vi "Drive_Execute.vi"() -> ()   [LabVIEW 2020]
uses:
  Drive_Control_States.ctl
  Drive_Cluster.ctl
  Drive_Orientation_States.ctl
  Globals/Drive_Globals.vi
  Globals/Sensor_Values.vi
  Globals/Calibration_And_Constant_Globals.vi
panel:
  in  "Back_Right_PID":T1(array[cluster])=[{"Kp"=0.0028, "Ki"=0.0, "Kd"=0.0, "N-Diff"=10, "N-Int"=10, "Int Error Window"=20.0, "Max Ouput"=0.5, "Min Output"=-0.5}, {"Kp"=0.0028, "Ki"=0.0, "Kd"=0.0, "N-Diff"=10, "N-Int"=10, "Int Error Window"=20.0, "Max Ouput"=0.5, "Min Output"=-0.5}]
  in  "Back_Left_PID":T1(array[cluster])=[{"Kp"=0.0028, "Ki"=0.0, "Kd"=0.0, "N-Diff"=10, "N-Int"=10, "Int Error Window"=20.0, "Max Ouput"=0.5, "Min Output"=-0.5}, {"Kp"=0.0028, "Ki"=0.0, "Kd"=0.0, "N-Diff"=10, "N-Int"=10, "Int Error Window"=20.0, "Max Ouput"=0.5, "Min Output"=-0.5}]
  in  "Front_Left_PID":T1(array[cluster])=[{"Kp"=0.0028, "Ki"=0.0, "Kd"=0.0, "N-Diff"=10, "N-Int"=10, "Int Error Window"=20.0, "Max Ouput"=0.5, "Min Output"=-0.5}, {"Kp"=0.0028, "Ki"=0.0, "Kd"=0.0, "N-Diff"=10, "N-Int"=10, "Int Error Window"=20.0, "Max Ouput"=0.5, "Min Output"=-0.5}]
  in  "Front_Right_PID":T1(array[cluster])=[{"Kp"=0.0028, "Ki"=0.0, "Kd"=0.0, "N-Diff"=10, "N-Int"=10, "Int Error Window"=20.0, "Max Ouput"=0.5, "Min Output"=-0.5}, {"Kp"=0.0028, "Ki"=0.0, "Kd"=0.0, "N-Diff"=10, "N-Int"=10, "Int Error Window"=20.0, "Max Ouput"=0.5, "Min Output"=-0.5}]
  out "angles":T2(graph)={"Front_Right"=176.5765625, "Front_ Left"=-4.482062499999984, "Back_Left"=-3.867593749999969, "Back_Right"=175.781515625}
  out "Front_Right":T3(graph)={"Command"=0.010270312500000017, "Proportional"=0.010270312500000017, "Integral"=0.0, "Derivative"=0.0, "Goal"=3.4234375000000057}
  out "Back_Right":T3(graph)={"Command"=0.01265545312500001, "Proportional"=0.01265545312500001, "Integral"=0.0, "Derivative"=0.0, "Goal"=4.218484375000003}
  out "Back_Left":T3(graph)={"Command"=0.011602781249999907, "Proportional"=0.011602781249999907, "Integral"=0.0, "Derivative"=0.0, "Goal"=3.867593749999969}
  out "Front_Left":T3(graph)={"Command"=0.013446187499999951, "Proportional"=0.013446187499999951, "Integral"=0.0, "Derivative"=0.0, "Goal"=4.482062499999984}
  in  "Manual_Target_Angle (deg)":dbl
  in  "Front_Panel_Control":bool
  in  "Hysteresis (deg)":dbl=10.0 format="%#_13g"
  # "0th index alpha,\n1st index beta"
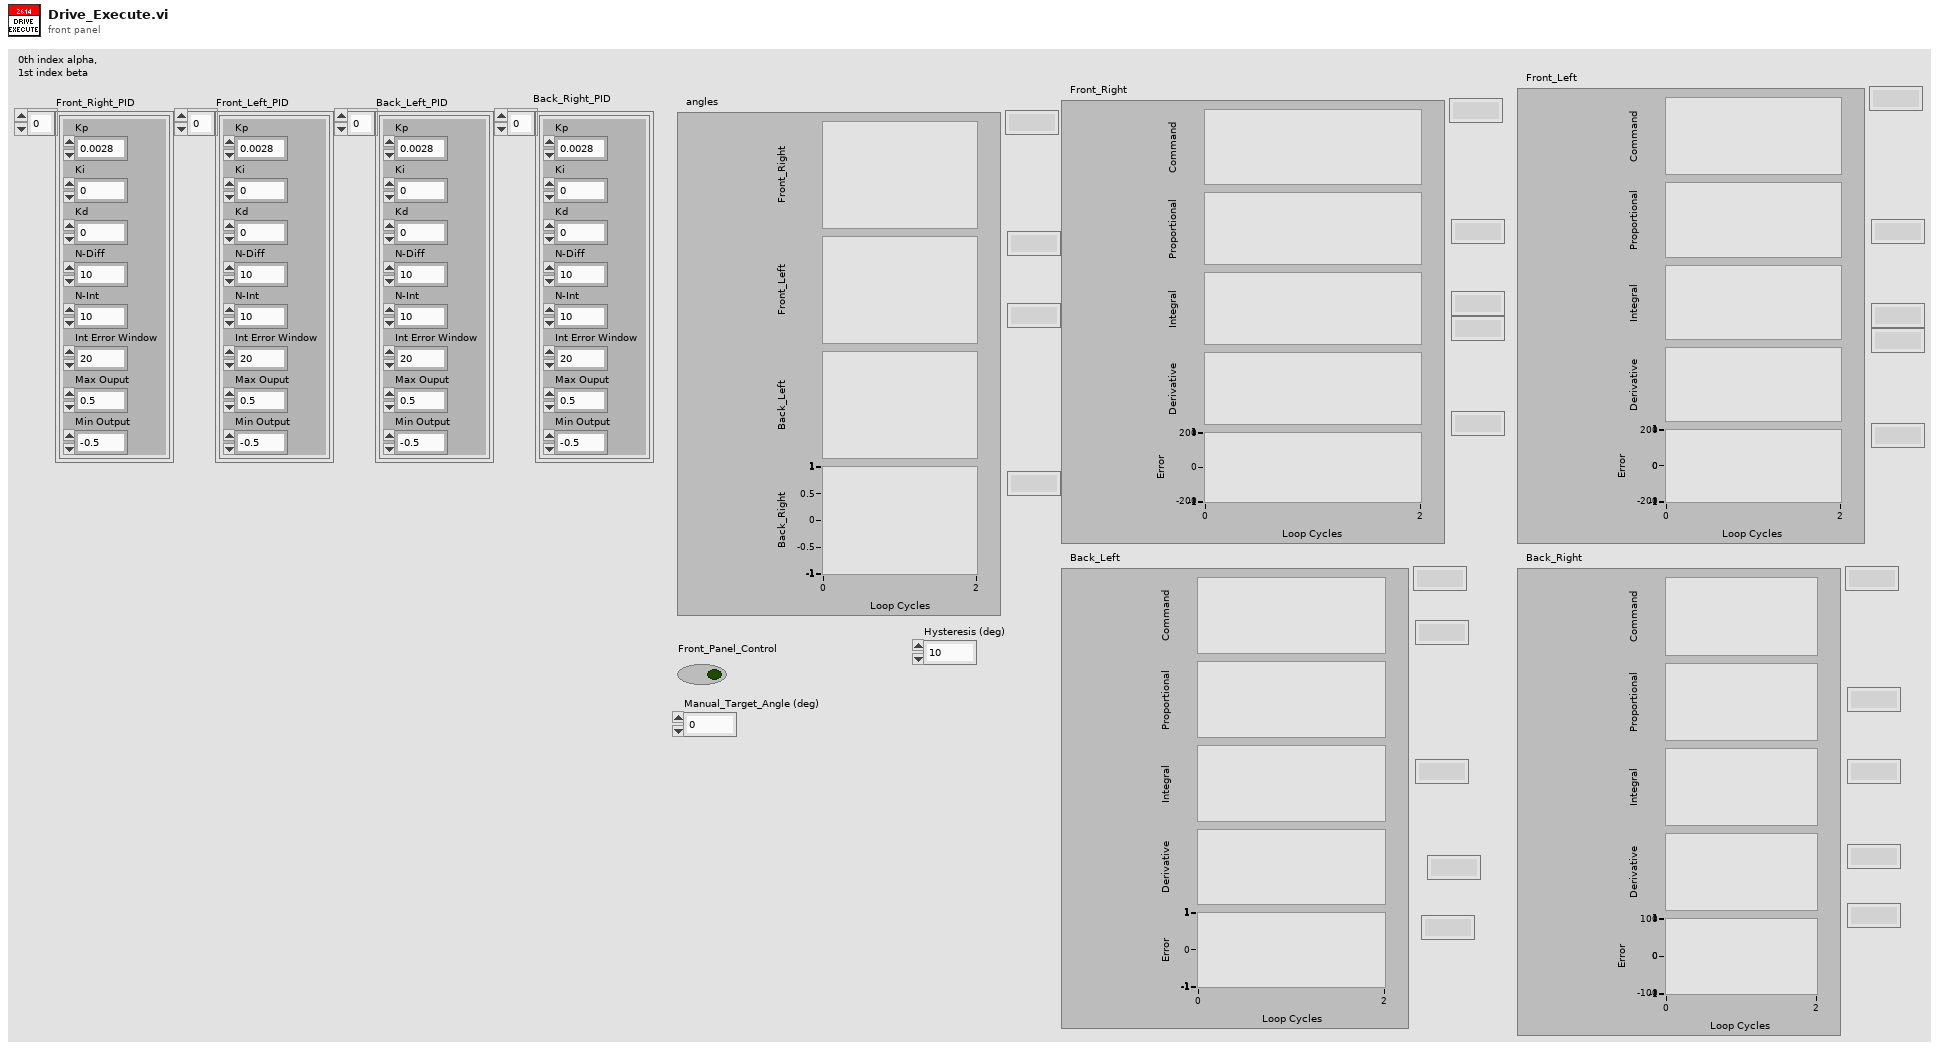
[diagram p1: front panel]
types:
  T1 = cluster{"Kp":dbl, "Ki":dbl, "Kd":dbl, "N-Diff":i32, "N-Int":i32, "Int Error Window":dbl, "Max Ouput":dbl, "Min Output":dbl}[]
  T2 = cluster{"Front_Right":dbl, "Front_ Left":dbl, "Back_Left":dbl, "Back_Right":dbl}
  T3 = cluster{"Command":dbl, "Proportional":dbl, "Integral":dbl, "Derivative":dbl, "Goal":dbl}
  T4 = typedef "Drive_Control_States.ctl" = enum16{"No-Op", "Manual_Control", "Command_DriveDistanceAtAngle", "Command_DrivePath", "Command_SetRobotPose", "Command_Rotate", "Go_To_X"}
  T5 = typedef "Drive_Cluster.ctl" = cluster{"Control_State":T4, "Vertical_Throttle":dbl, "Lateral_Throttle":dbl, "Rotational_Throttle":dbl, "Strafe_In_Deadband":bool, "Rotation_In_Deadband":bool, "Orientation_State":T6, "Parameters":dbl[], "Step":i32, "Auto_Notifier":refnum<notifier>, "PathName":string}
  T6 = typedef "Drive_Orientation_States.ctl" = enum16{"Robot-Oriented", "Field-Oriented"}
  T7 = cluster{"Kp":dbl, "Ki":dbl, "Kd":dbl, "N-Diff":i32, "N-Int":i32, "Int Error Window":dbl, "Max Ouput":dbl, "Min Output":dbl}
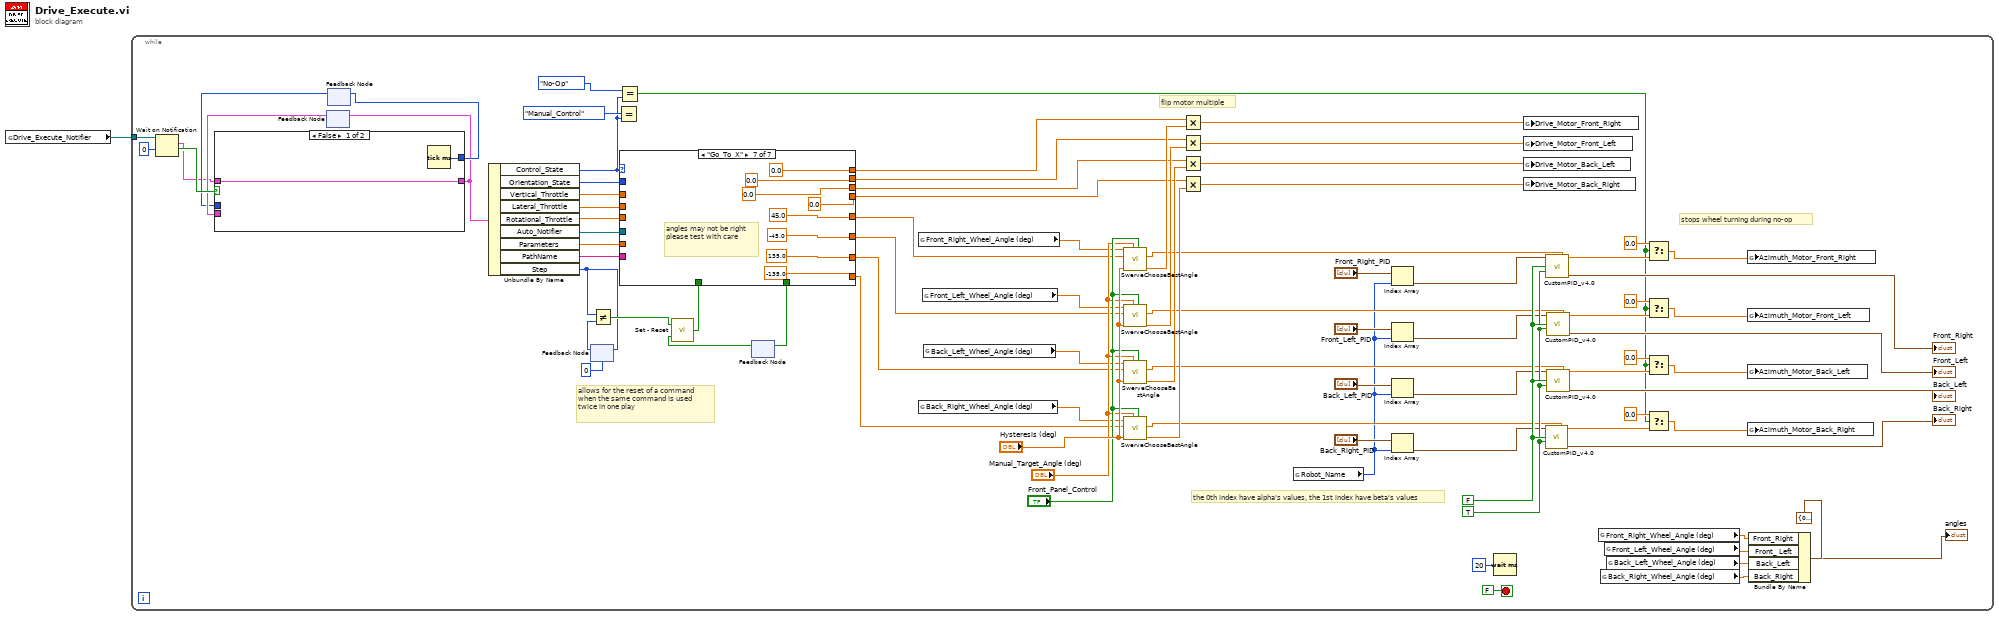
[diagram p0: block diagram]
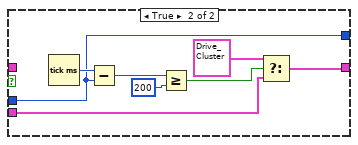
[diagram p2: hidden frame]
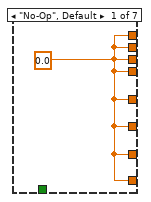
[diagram p3: hidden frame]
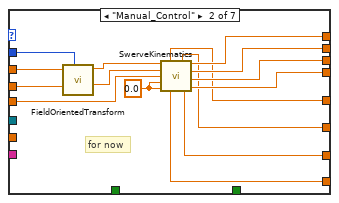
[diagram p4: hidden frame]
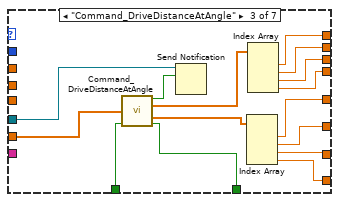
[diagram p5: hidden frame]
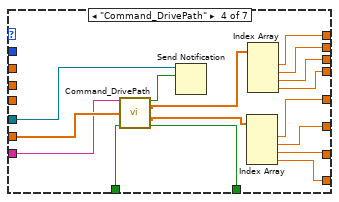
[diagram p6: hidden frame]
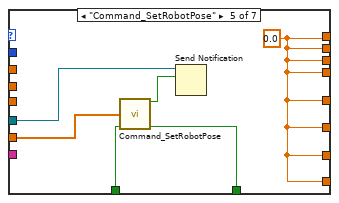
[diagram p7: hidden frame]
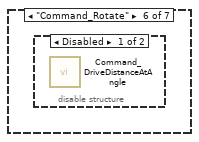
[diagram p8: hidden frame]
diagram:
  n1 = global read "Drive_Globals.vi" "Drive_Execute_Notifier"() -> (w1:refnum<notifier>)
  n2 = while {
    tunnel: w1 -> [w87]
    stop <- FALSE stop-if-true
    w85 = TRUE
    w86 = FALSE
    # "the 0th index have alpha's values, the 1st index have beta's values"
    # "stops wheel turning during no-op"
    # "flip motor multiple"
    # "allows for the reset of a command when the same command is used twice in one play"
    n3 = Wait on Notification(notifier=w87, timeout in ms (-1)=0) -> (notification=w4:T5, timed out?=w32:bool)  [unwired: 2 in, 2 out]
    n4 = feedback #1() -> (w7:T5)  [unwired: 1 in]
    n5 = feedback #2() -> (w5:u32)  [unwired: 1 in]
    n6 = case shown="False" w32 {
      tunnel: w4 -> [w91 _]
      tunnel: [w91 w99] -> w3
      tunnel: w7 -> [_ w98]
      tunnel: [w90 w96] -> w6
      tunnel: w5 -> [_ w96]
      frame False {
        n7 = Tick Count (ms)() -> (millisecond timer value=w90:u32)
      }
      frame True {
        n8 = Tick Count (ms)() -> (millisecond timer value=w97:u32)
        n9 = Subtract(x=w97, y=w96) -> (x-y=w94:u32)
        n10 = Greater Or Equal?(x=w94, y=u32 200) -> (x >= y?=w95:bool)
        n11 = Select(t=T5 {"Control_State"=enum."Manual_Control", "Vertical_Throttle"=0.0, "Lateral_Throttle"=0.0, "Rotational_Throttle"=0.0, "Strafe_In_Deadband"=FALSE, "Rotation_In_Deadband"=FALSE, "Orientation_State"=enum."Robot-Oriented", "Parameters"=[], "Step"=0, "Auto_Notifier"=refnum, "PathName"=""} ("Cluster"), s=w95, f=w98) -> (s? t:f=w99:T5)
      }
    }
    n12 = feedback-in #1(w3) -> ()
    n13 = feedback-in #2(w6) -> ()
    n14 = Unbundle By Name(w3) -> ("Control_State"=w26:T4, "Orientation_State"=w2:T6, "Vertical_Throttle"=w72:dbl, "Lateral_Throttle"=w71:dbl, "Rotational_Throttle"=w79:dbl, "Auto_Notifier"=w61:refnum<notifier>, "Parameters"=w60:dbl[], "PathName"=w20:string, "Step"=w21:i32)
    n15 = feedback-in #3(w21) -> ()
    n16 = feedback #3(0 ("Step")) -> (w59:i32)
    n17 = Not Equal?(x=w21, y=w59) -> (x != y?=w30:bool)
    n18 = Equal?(x=Drive_Control_States."Manual_Control" ("Control_State"), y=w26) -> ()  [unwired: 1 out]
    n19 = Equal?(x=Drive_Control_States."No-Op", y=w26) -> (x = y?=w37:bool)
    n20 = feedback #4() -> (w29:bool)  [unwired: 1 in]
    n21 = call "Set - Reset.vi"("Reset"=w29, "Set"=w30) -> ("Output"=w28:bool)
    n22 = case shown="\"Go_To_X\"" w26 {
      tunnel: [w100 w111 w126 w145 w147 _ 0.0 ("Numeric")] -> w52
      tunnel: [w100 w110 w125 w144 w147 _ 0.0 ("Numeric")] -> w51
      tunnel: [w100 w109 w124 w143 w147 _ 0.0 ("Numeric")] -> w50
      tunnel: [w100 w108 w123 w142 w147 _ 0.0 ("Numeric")] -> w49
      tunnel: [w100 w107 w121 w141 w147 _ 45.0 ("Numeric")] -> w56
      tunnel: [w100 w106 w120 w140 w147 _ -45.0 ("Numeric")] -> w55
      tunnel: [w100 w105 w119 w139 w147 _ 135.0 ("Numeric")] -> w54
      tunnel: [w100 w104 w118 w138 w147 _ -135.0 ("Numeric")] -> w53
      tunnel: w79 -> [_ w113 _ _ _ _ _]
      tunnel: w2 -> [_ w101 _ _ _ _ _]
      tunnel: w72 -> [_ w102 _ _ _ _ _]
      tunnel: w71 -> [_ w103 _ _ _ _ _]
      tunnel: w61 -> [_ _ w129 w146 w152 _ _]
      tunnel: w60 -> [_ _ w130 w136 w150 _ _]
      tunnel: w28 -> [_ _ w117 w137 w151 _ _]
      tunnel: [_ _ w116 w132 w148 _ _] -> w31
      tunnel: w20 -> [_ _ _ w131 _ _ _]
      frame "No-Op", Default {
        w100 = 0.0 ("Numeric")
      }
      frame "Manual_Control" {
        w112 = 0.0 ("Cx (in)")
        # "for now"
        n23 = call "FieldOrientedTransform.vi"("Orientation Mode"=w101, "Joystick Y"=w103, "Joystick X"=w102) -> ("Joystick Y'"=w114:dbl, "Joystick X'"=w115:dbl)  [unwired: 7 in]
        n24 = call "SwerveKinematics.vi"("Joystick X"=w115, "Joystick Y"=w114, "Joystick Rotation"=w113, "Cx (in)"=w112, "Cy (in)"=w112) -> ("Module 0 Angle (deg)"=w107:dbl, "Module 1 Angle (deg)"=w106:dbl, "Module 0 Velocity Command (ul)"=w111:dbl, "Module 1 Velocity Command (ul)"=w110:dbl, "Module 2 Velocity Command (ul)"=w109:dbl, "Module 3 Angle (deg)"=w104:dbl, "Module 2 Angle (deg)"=w105:dbl, "Module 3 Velocity Command (ul)"=w108:dbl)  [unwired: 3 in]
      }
      frame "Command_DriveDistanceAtAngle" {
        n25 = call "Command_DriveDistanceAtAngle.vi"("Parameters"=w130, "Startup"=w117) -> ("Completed"=w128:bool, "Target_Drive_Powers"=w127:dbl[], "Target_Wheel_Angles"=w122:dbl[], "Reinit"=w116:bool)  [unwired: 10 in]
        n26 = Send Notification(notification=w128, notifier=w129) -> ()  [unwired: 1 in, 2 out]
        n27 = Index Array(array=w122) -> (element #1=w121:dbl, element #2=w120:dbl, element #3=w119:dbl, element #4=w118:dbl)  [unwired: 4 in]
        n28 = Index Array(array=w127) -> (element #1=w126:dbl, element #2=w125:dbl, element #3=w124:dbl, element #4=w123:dbl)  [unwired: 4 in]
      }
      frame "Command_DrivePath" {
        n29 = call "Command_DrivePath.vi"("Name of Path"=w131, "Parameters"=w136, "Startup"=w137) -> ("Completed"=w133:bool, "Drive_Motor_Values"=w135:dbl[], "Azimuth_Motor_Values"=w134:dbl[], "Reinit"=w132:bool)  [unwired: 9 in]
        n30 = Send Notification(notification=w133, notifier=w146) -> ()  [unwired: 1 in, 2 out]
        n31 = Index Array(array=w134) -> (element #1=w141:dbl, element #2=w140:dbl, element #3=w139:dbl, element #4=w138:dbl)  [unwired: 4 in]
        n32 = Index Array(array=w135) -> (element #1=w145:dbl, element #2=w144:dbl, element #3=w143:dbl, element #4=w142:dbl)  [unwired: 4 in]
      }
      frame "Command_SetRobotPose" {
        w147 = 0.0 ("Numeric")
        n33 = call "Command_SetRobotPose.vi"("Parameters"=w150, "Startup"=w151) -> ("Completed"=w149:bool, "Reinit"=w148:bool)  [unwired: 12 in]
        n34 = Send Notification(notification=w149, notifier=w152) -> ()  [unwired: 1 in, 2 out]
      }
      frame "Command_Rotate" {
        n35 = disable-structure shown="Disabled" {
          frame Disabled {
            n36 = call "Command_DriveDistanceAtAngle.vi"() -> ()  [unwired: 12 in, 4 out]
          }
          frame Enabled {
          }
        }
      }
      frame "Go_To_X" {
        # "angles may not be right\nplease test with care"
      }
    }
    n37 = feedback-in #4(w31) -> ()
    n38 = global read "Sensor_Values.vi" "Front_Right_Wheel_Angle (deg)"() -> (w57:dbl)
    n39 = global read "Sensor_Values.vi" "Back_Right_Wheel_Angle (deg)"() -> (w66:dbl)
    n40 = global read "Sensor_Values.vi" "Front_Left_Wheel_Angle (deg)"() -> (w68:dbl)
    n41 = global read "Sensor_Values.vi" "Back_Left_Wheel_Angle (deg)"() -> (w67:dbl)
    n42 = call "SwerveChooseBestAngle.vi"("Goal Override"="Front_Panel_Control", "Goal Override Angle (deg) [-180,+180]"="Manual_Target_Angle (deg)", "Hysteresis (deg)"="Hysteresis (deg)", "Goal Angle (deg) [-180,+180]"=w56, "Current Angle (deg) [-180,+180]"=w57) -> ("Flip Drive Motor Multiple"=w83:dbl, "Angular Distance (deg)"=w25:dbl)  [unwired: 5 in]
    n43 = call "SwerveChooseBestAngle.vi"("Goal Override"="Front_Panel_Control", "Goal Override Angle (deg) [-180,+180]"="Manual_Target_Angle (deg)", "Hysteresis (deg)"="Hysteresis (deg)", "Goal Angle (deg) [-180,+180]"=w55, "Current Angle (deg) [-180,+180]"=w68) -> ("Flip Drive Motor Multiple"=w82:dbl, "Angular Distance (deg)"=w24:dbl)  [unwired: 5 in]
    n44 = call "SwerveChooseBestAngle.vi"("Goal Override"="Front_Panel_Control", "Goal Override Angle (deg) [-180,+180]"="Manual_Target_Angle (deg)", "Hysteresis (deg)"="Hysteresis (deg)", "Goal Angle (deg) [-180,+180]"=w54, "Current Angle (deg) [-180,+180]"=w67) -> ("Flip Drive Motor Multiple"=w81:dbl, "Angular Distance (deg)"=w23:dbl)  [unwired: 5 in]
    n45 = call "SwerveChooseBestAngle.vi"("Goal Override"="Front_Panel_Control", "Goal Override Angle (deg) [-180,+180]"="Manual_Target_Angle (deg)", "Hysteresis (deg)"="Hysteresis (deg)", "Goal Angle (deg) [-180,+180]"=w53, "Current Angle (deg) [-180,+180]"=w66) -> ("Flip Drive Motor Multiple"=w80:dbl, "Angular Distance (deg)"=w22:dbl)  [unwired: 5 in]
    n46 = Multiply(x=w52, y=w83) -> (x*y=w48:dbl)
    n47 = Multiply(x=w51, y=w82) -> (x*y=w47:dbl)
    n48 = Multiply(x=w50, y=w81) -> (x*y=w18:dbl)
    n49 = Multiply(x=w49, y=w80) -> (x*y=w46:dbl)
    n50 = global read "Calibration_And_Constant_Globals.vi" "Robot_Name"() -> (w13:enum16{"Alpha-2022", "Beta-2022"})
    n51 = Index Array(array="Front_Right_PID", index=w13) -> (element=w12:T7)
    n52 = Index Array(array="Front_Left_PID", index=w13) -> (element=w11:T7)
    n53 = Index Array(array="Back_Left_PID", index=w13) -> (element=w10:T7)
    n54 = Index Array(array="Back_Right_PID", index=w13) -> (element=w9:T7)
    n55 = Wait (ms)(milliseconds to wait=u32 20) -> ()  [unwired: 1 out]
    n56 = global write "Drive_Globals.vi" "Drive_Motor_Front_Right"(w48) -> ()
    n57 = global write "Drive_Globals.vi" "Drive_Motor_Front_Left"(w47) -> ()
    n58 = global write "Drive_Globals.vi" "Drive_Motor_Back_Left"(w18) -> ()
    n59 = global write "Drive_Globals.vi" "Drive_Motor_Back_Right"(w46) -> ()
    n60 = call "CustomPID_v4.0.vi"("PID Tuning Parameters"=w9, "Custom Error Calculation"=w22, "Reset on Goal Change ?"=w86, "Use Custom Error Calculation ?"=w85) -> ("Command"=w45:dbl, "Controller Summary"=→"Back_Right":T3)  [unwired: 8 in, 2 out]
    n61 = call "CustomPID_v4.0.vi"("PID Tuning Parameters"=w12, "Custom Error Calculation"=w25, "Reset on Goal Change ?"=w86, "Use Custom Error Calculation ?"=w85) -> ("Command"=w38:dbl, "Controller Summary"=→"Front_Right":T3)  [unwired: 8 in, 2 out]
    n62 = call "CustomPID_v4.0.vi"("PID Tuning Parameters"=w11, "Custom Error Calculation"=w24, "Reset on Goal Change ?"=w86, "Use Custom Error Calculation ?"=w85) -> ("Command"=w39:dbl, "Controller Summary"=→"Front_Left":T3)  [unwired: 8 in, 2 out]
    n63 = call "CustomPID_v4.0.vi"("PID Tuning Parameters"=w10, "Custom Error Calculation"=w23, "Reset on Goal Change ?"=w86, "Use Custom Error Calculation ?"=w85) -> ("Command"=w40:dbl, "Controller Summary"=→"Back_Left":T3)  [unwired: 8 in, 2 out]
    n64 = global read "Sensor_Values.vi" "Front_Right_Wheel_Angle (deg)"() -> (w62:dbl)
    n65 = global read "Sensor_Values.vi" "Back_Right_Wheel_Angle (deg)"() -> (w63:dbl)
    n66 = global read "Sensor_Values.vi" "Front_Left_Wheel_Angle (deg)"() -> (w65:dbl)
    n67 = global read "Sensor_Values.vi" "Back_Left_Wheel_Angle (deg)"() -> (w64:dbl)
    n68 = Select(t=0.0, s=w37, f=w38) -> (s? t:f=w36:dbl)
    n69 = Select(t=0.0, s=w37, f=w39) -> (s? t:f=w35:dbl)
    n70 = Select(t=0.0, s=w37, f=w40) -> (s? t:f=w19:dbl)
    n71 = Select(t=0.0, s=w37, f=w45) -> (s? t:f=w34:dbl)
    n72 = global write "Drive_Globals.vi" "Azimuth_Motor_Front_Right"(w36) -> ()
    n73 = global write "Drive_Globals.vi" "Azimuth_Motor_Front_Left"(w35) -> ()
    n74 = global write "Drive_Globals.vi" "Azimuth_Motor_Back_Left"(w19) -> ()
    n75 = global write "Drive_Globals.vi" "Azimuth_Motor_Back_Right"(w34) -> ()
    n76 = Bundle By Name(cluster=T2 {"Front_Right"=0.0, "Front_ Left"=0.0, "Back_Left"=0.0, "Back_Right"=0.0}, "Front_Right"=w62, "Front_ Left"=w65, "Back_Left"=w64, "Back_Right"=w63) -> (→"angles":T2)
  }
